vi "Process.vi"(8 "error in":errorcluster, 11 "MAUI":refnum<class "MAUI.lvclass">) -> (0 "error out":errorcluster, 3 "MAUI out":refnum<class "MAUI.lvclass">)   [LabVIEW 2016, in "MAUI.lvclass"]
doc: "---------------------------------------------------------------\nJKI State Machine Objects™\nhttp://jki.net/state-machine-objects/\nCopyright (C) 2005-2015, JKI <info@jki.net>\nALL RIGHTS RESERVEDJKI State Machine Objects (SMO) 1.0.0.5\nJKI - JKI\nCopyright (c) 2016, JKI"
uses:
  MAUI.lvclass
  C:/Program Files (x86)/National Instruments/LabVIEW 2016/vi.lib/JKI/JKI SMO/SMO/SMO.lvclass
  C:/Program Files (x86)/National Instruments/LabVIEW 2016/vi.lib/JKI/JKI SMO/SMO.UI/SMO.UI.lvclass
  <vilib>/JKI/JKI SMO/SMO/Typedefs/Parent Call--Enum.ctl
  MAUI.lvclass/MAUI.ctl
  <vilib>/JKI/JKI SMO/SMO.UI/SMO.UI.lvclass
  <vilib>/JKI/JKI SMO/SMO/SMO.lvclass
panel:
  # "For instructions on how to use the JKI State Machine Objects, examples and video tutorials, visit:\nhttp://jki.net/state-machine-objects/\n\nJKI State Machine Objects™\nhttp://jki.net/state-machine-objects/\nCopyright (C) 2005-2015, JKI <info@jki.net>\nALL RIGHTS RESERVED"
  # "SMO UI Template"
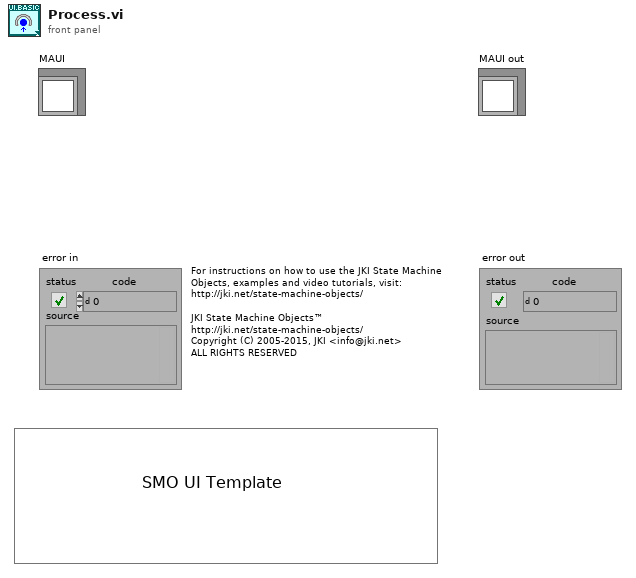
[diagram p1: front panel]
types:
  T1 = typedef "SMO.lvclass/Parent Call--Enum.ctl" = enum16{"Allows parent to run", "Does not request parent to run"}
  T2 = enum32{"invalid app kind", "Development System", "Run Time System", "Student Edition", "Embedded LabVIEW", "Evaluation", "Custom"}
  T3 = enum32{"Invalid", "Standard", "Closed", "Hidden", "Minimized", "Maximized"}
  T4 = typedef "MAUI.lvclass/PrivateEvents--MAUI.Update Left Subpanel.ctl" = i32
  T5 = cluster{"Core":cluster{"Current VI Reference":refnum<vi>, "Close Panel on Exit?":bool, "error":errorcluster}, "Self Reference":refnum<class "MAUI.lvclass">, "Your string data":string}
  T6 = typedef "MAUI.lvclass/PrivateEvents--MAUI.UpdateRightSubpanel.ctl" = i32
  T7 = typedef "MAUI.lvclass/PanelData.ctl" = cluster{"Subpanel":refnum<vi>, "Ring":refnum<vi>, "Active":i32}
  T8 = typedef "MAUI.lvclass/PanelDataNotifier.ctl" = refnum<notifier>
  T9 = cluster{"Subpanel":refnum<vi>, "Ring":refnum<vi>, "Active":i32}
  T10 = cluster{"Current VI Reference":refnum<vi>, "Close Panel on Exit?":bool, "error":errorcluster}
  T11 = typedef "SMO.lvclass/Protected Events.ctl" = cluster{"StopProcesses":refnum<user-event>, "AbortProcesses":refnum<user-event>, "Config Changed":refnum<user-event>, "Dependency":refnum<user-event>}
  T12 = typedef "MAUI.lvclass/PrivateEvents--Cluster.ctl" = cluster{"SetLeftData":refnum<user-event>, "SetRightData":refnum<user-event>, "GetRightData":refnum<user-event>, "GetLeftData":refnum<user-event>, "SetEmbedded":refnum<user-event>, "GetEmbedded":refnum<user-event>, "Update Left Subpanel":refnum<user-event>, "UpdateRightSubpanel":refnum<user-event>}
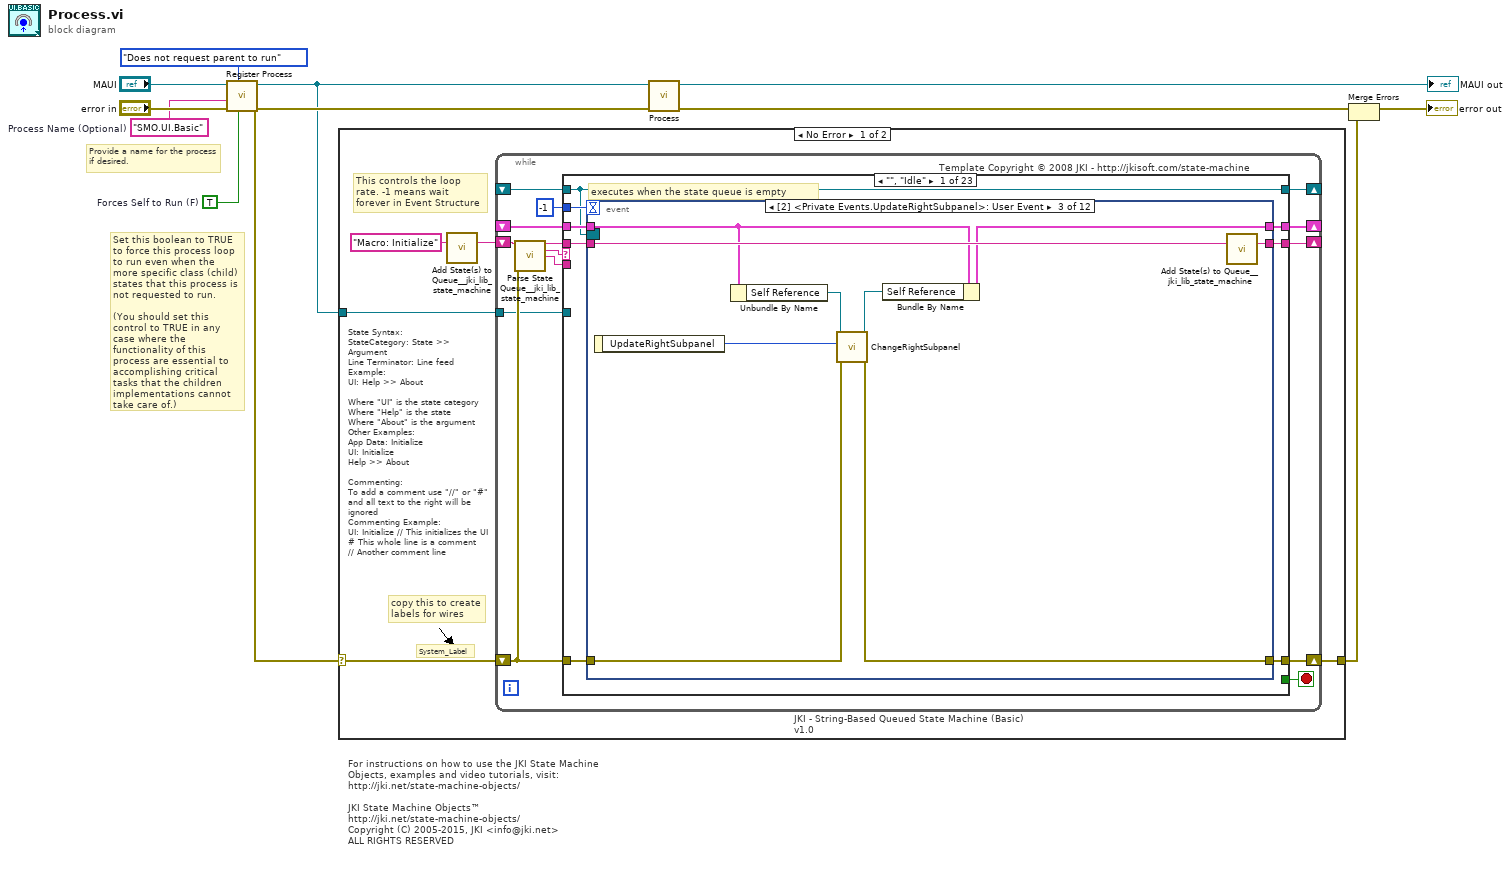
[diagram p0: block diagram]
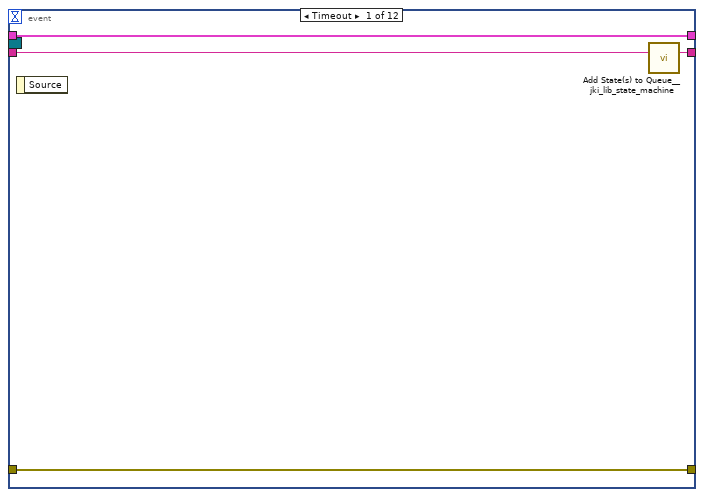
[diagram p2: hidden frame]
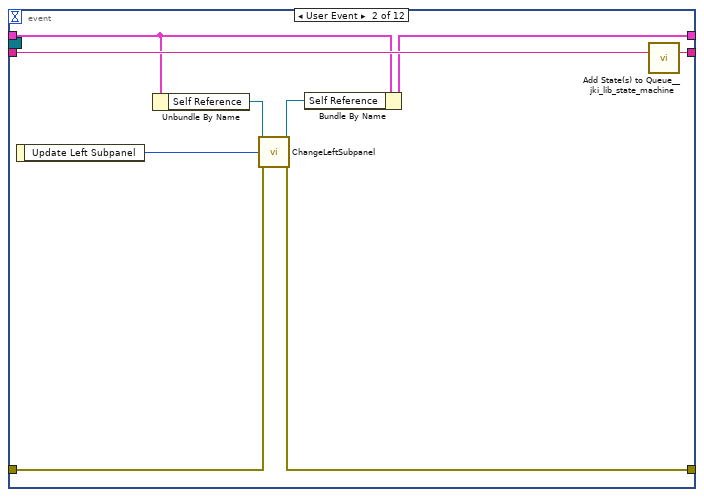
[diagram p3: hidden frame]
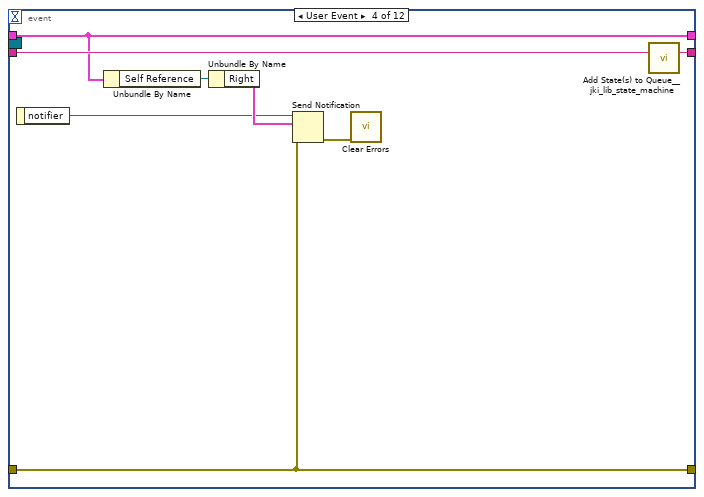
[diagram p4: hidden frame]
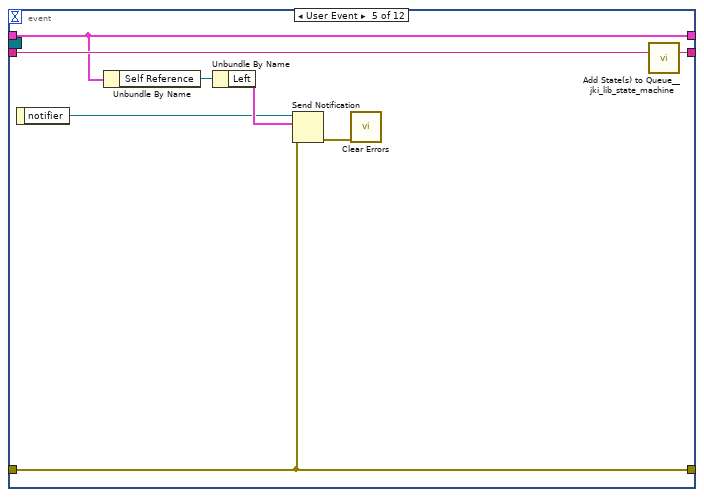
[diagram p5: hidden frame]
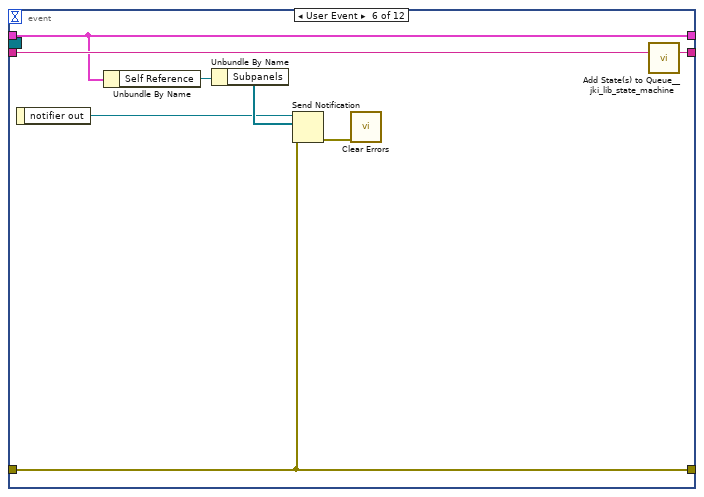
[diagram p6: hidden frame]
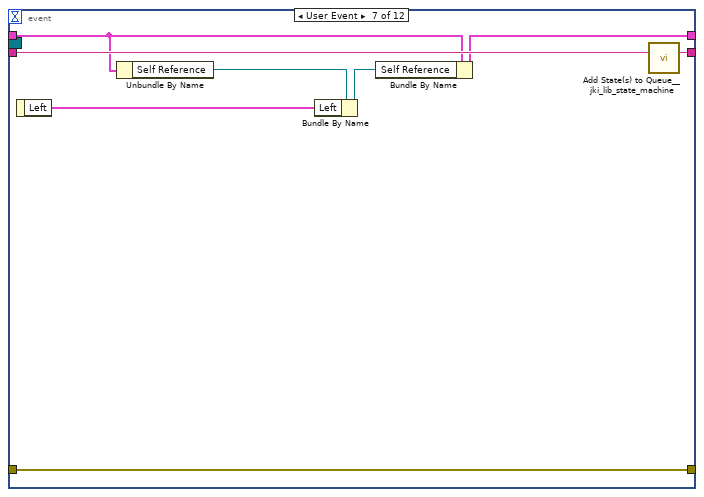
[diagram p7: hidden frame]
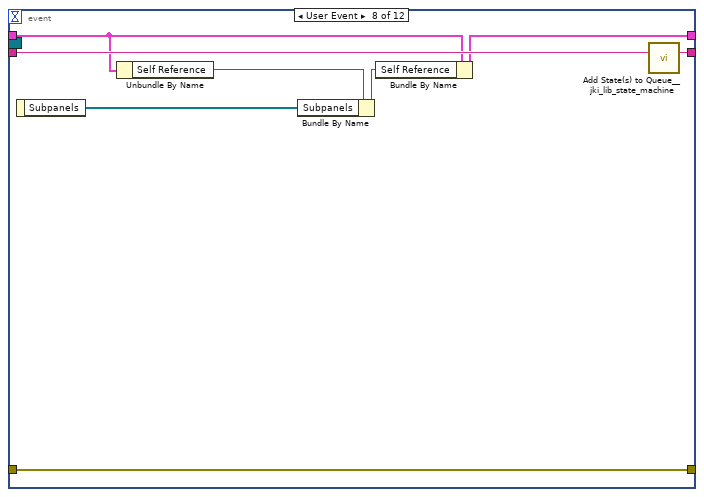
[diagram p8: hidden frame]
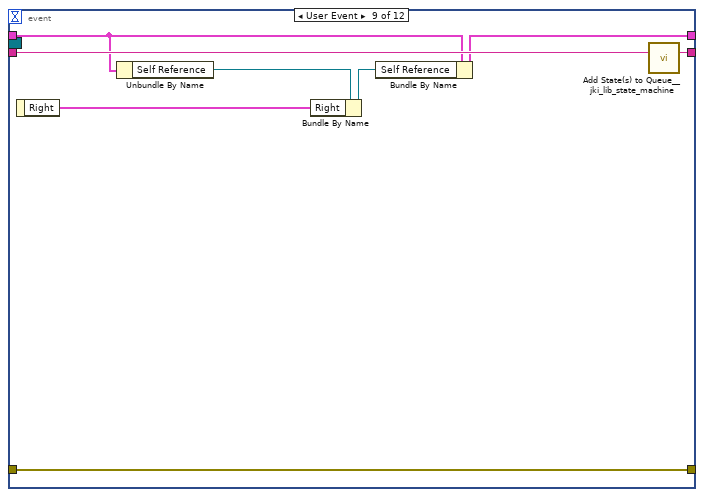
[diagram p9: hidden frame]
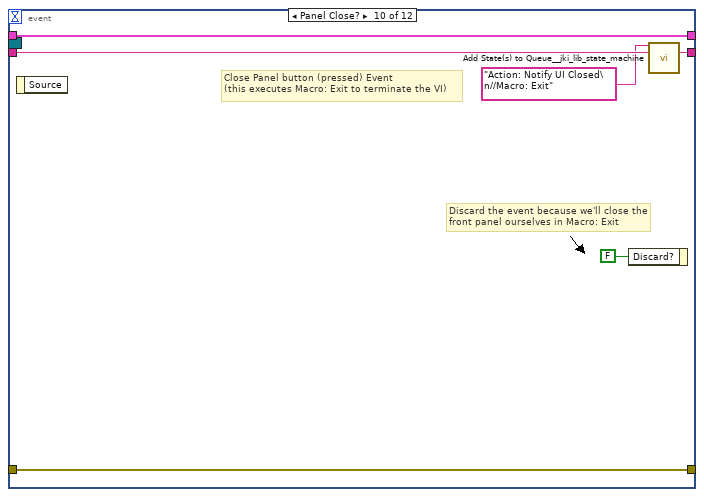
[diagram p10: hidden frame]
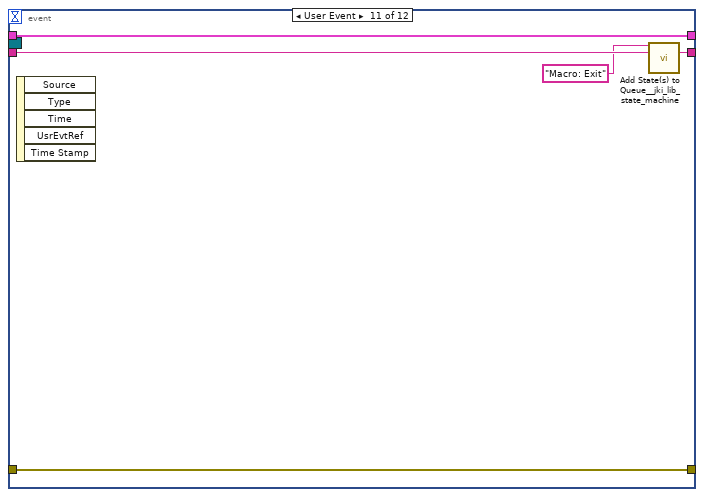
[diagram p11: hidden frame]
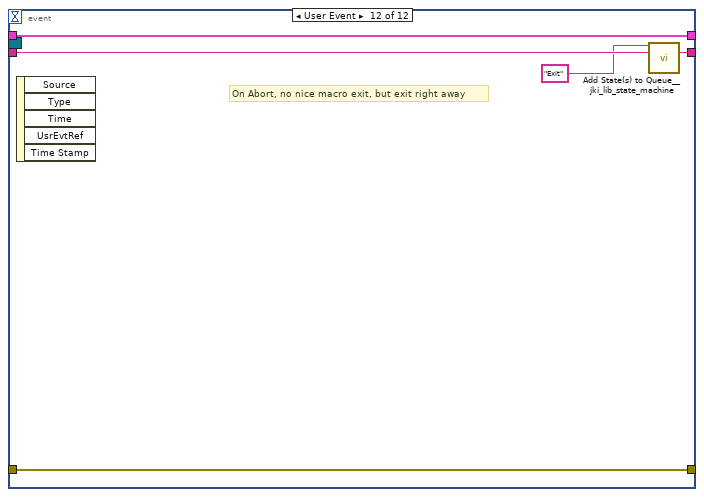
[diagram p12: hidden frame]
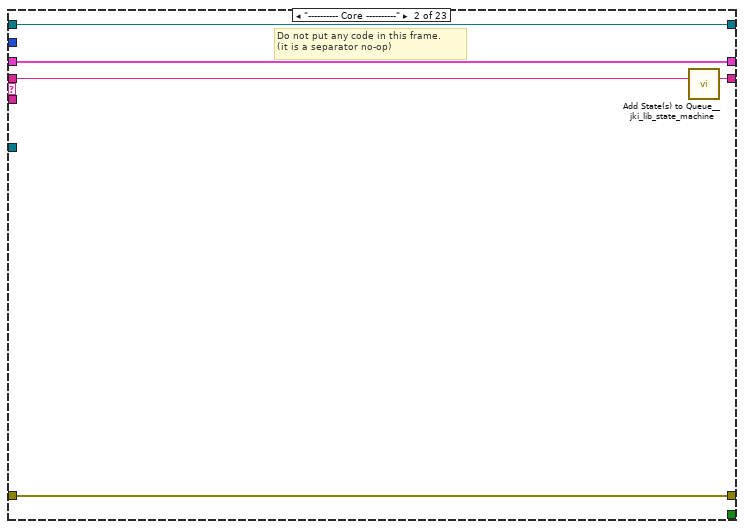
[diagram p13: hidden frame]
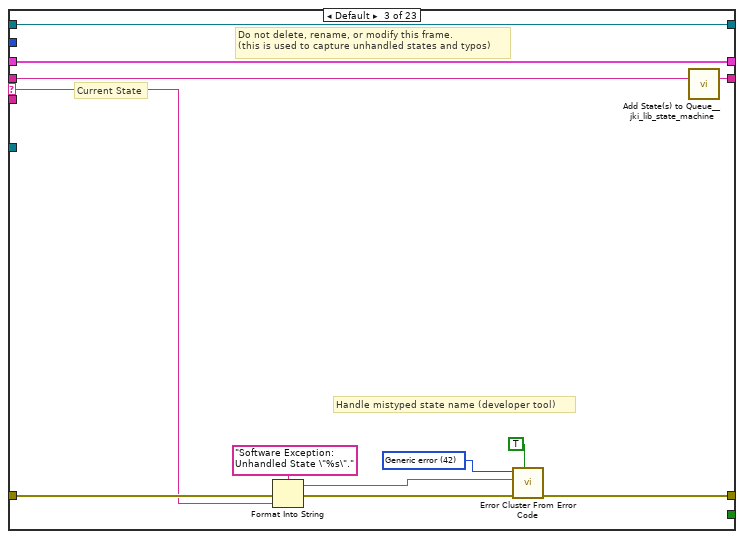
[diagram p14: hidden frame]
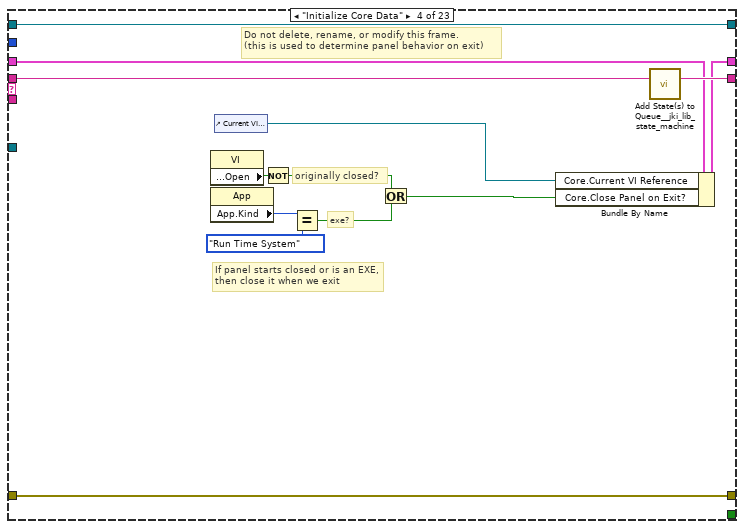
[diagram p15: hidden frame]
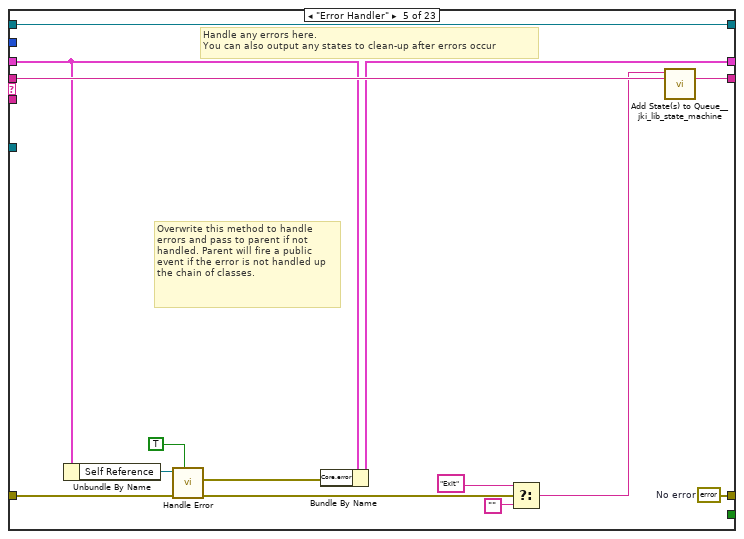
[diagram p16: hidden frame]
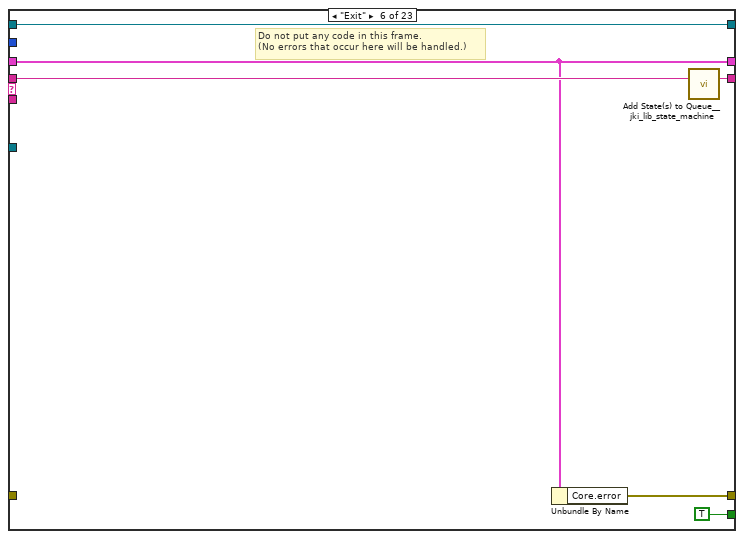
[diagram p17: hidden frame]
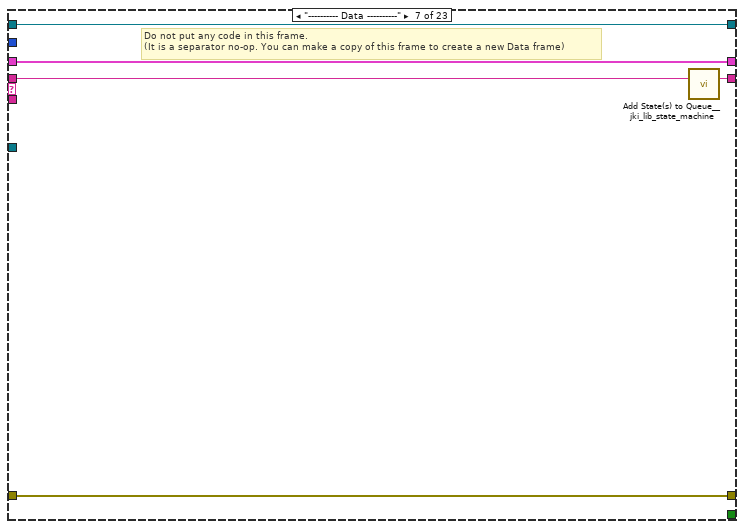
[diagram p18: hidden frame]
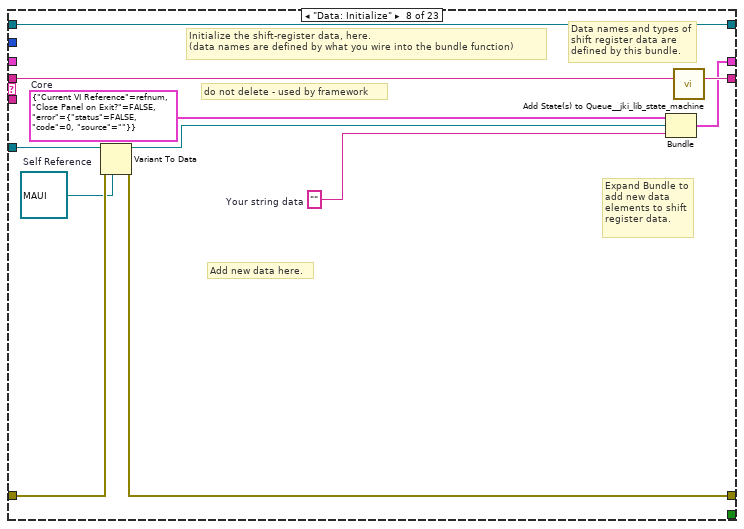
[diagram p19: hidden frame]
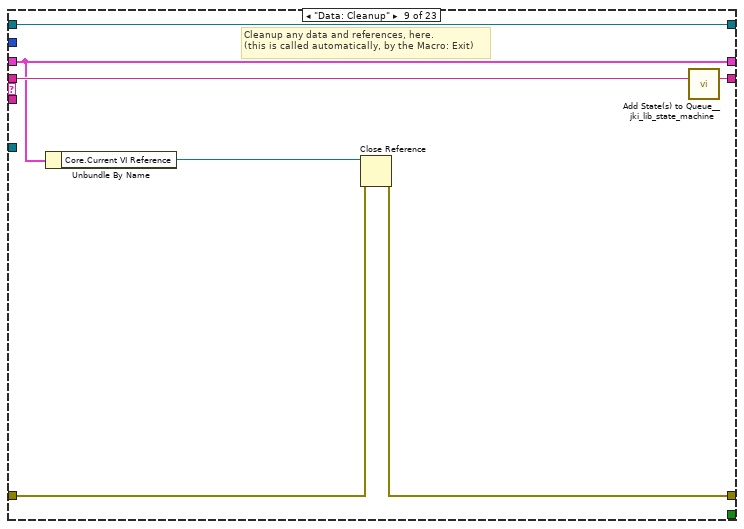
[diagram p20: hidden frame]
diagram:
  w2 = TRUE  # Forces Self to Run (F)
  w1 = "SMO.UI.Basic"  # Process Name (Optional)
  # "Provide a name for the process\nif desired."
  # "Set this boolean to TRUE to force this process loop to run even when the more specific class (child) states that this process is not requested to run.\n\n(You should set this control to TRUE in any case where the functionality of this process are essential to accomplishing critical tasks that the children implementations cannot take care of.)"
  # "For instructions on how to use the JKI State Machine Objects, examples and video tutorials, visit:\nhttp://jki.net/state-machine-objects/\n\nJKI State Machine Objects™\nhttp://jki.net/state-machine-objects/\nCopyright (C) 2005-2015, JKI <info@jki.net>\nALL RIGHTS RESERVED"
  n1 = call <vilib>:"Register Process.vi"("Forces Self to Run (F)"=w2, "Parent Call"=Parent_Call--Enum."Does not request parent to run", "error in (no error)"="error in", "Process Name (optional)"=w1, "SMO"="MAUI") -> ("error out"=w8:errorcluster, "SMO out"=w7:refnum<class "MAUI.lvclass">)  [unwired: 5 in]
  n2 = case shown="No Error" w8 {
    selector: w8 -> [w13 w339]
    tunnel: w7 -> [w14 _]
    tunnel: [w12 w339] -> w4
    frame No Error {
      # "State Syntax:\nStateCategory: State >> Argument\nLine Terminator: Line feed\nExample:\nUI: Help >> About\n\nWhere \"UI\" is the state category\nWhere \"Help\" is the state\nWhere \"About\" is the argument\nOther Examples:\nApp Data: Initialize\nUI: Initialize\nHelp >> About\n\nCommenting:\nTo add a comment use \"//\" or \"#\" and all text to the right will be ignored\nCommenting Example:\nUI: Initialize // This initializes the UI\n# This whole line is a comment\n// Another comment line"
      # "copy this to create labels for wires"
      # "This controls the loop rate. -1 means wait forever in Event Structure"
      # "System_Label"
      n3 = call <vilib>:"Add State(s) to Queue__jki_lib_state_machine.vi"("State(s) in (\"\")"="Macro: Initialize") -> ("States Out"=w16:string)  [unwired: 14 in]
      n4 = while "JKI - String-Based Queued State Machine (Basic) v1.0" {
        shift-right: [w23] -> _
        shift-left: _ -> [w22]
        shift-right: [w26] -> w12
        shift-left: w13 -> [w20]
        shift-right: [w25] -> _
        shift-left: w16 -> [w27]
        tunnel: w14 -> [w19]
        shift-right: [w18] -> _
        shift-left: _ -> [w17]
        stop <- w24 stop-if-true
        # "Template Copyright © 2008 JKI - http://jkisoft.com/state-machine"
        n5 = call <vilib>:"Parse State Queue__jki_lib_state_machine.vi"("State Queue"=w27, "Error In (no error)"=w20) -> ("Remaining States"=w29:string, "Current State"=w30:string, "Arguments"=w28:string)  [unwired: 11 in]
        n6 = case shown="\"\", \"Idle\"" w30 {
          selector: w30 -> [_ _ w131 _ _ _ _ _ _ _ _ _ _ _ _ _ _ _ _ _ _ _ _]
          tunnel: w29 -> [w38 w129 w135 w154 w168 w174 w179 w190 w197 w202 w207 w214 w230 w262 w271 w285 w290 w301 w306 w318 w324 w331 w338]
          tunnel: w28 -> [_ _ _ _ _ _ _ _ _ _ _ w208 w224 _ _ _ _ _ _ _ _ _ _]
          tunnel: w22 -> [w36 w126 w133 w145 w157 w170 w176 _ w192 w199 w205 w212 w226 w259 w267 w276 w287 w298 w303 w316 w322 w327 w334]
          tunnel: [w35 w127 w137 w151 w159 w169 w177 w185 w193 w200 w204 w209 w227 w260 w269 w283 w288 w292 w304 w311 w319 w328 w332] -> w26
          tunnel: w20 -> [w34 w127 w136 w151 w164 _ w177 w186 w194 w200 w204 w210 w228 w260 w269 w283 w288 w293 w304 w313 w320 w328 w333]
          tunnel: [w37 w128 w134 w153 w167 w173 w178 w189 w196 w201 w206 w213 w229 w261 w270 w284 w289 w300 w305 w317 w323 w330 w337] -> w25
          tunnel: [_ _ _ _ _ TRUE _ _ _ _ _ _ _ _ _ _ _ _ _ _ _ _ _] -> w24
          tunnel: [w33 w126 w133 w152 w156 w170 w176 w188 w192 w199 w205 w212 w226 w259 w267 w276 w287 w298 w303 w316 w322 w326 w334] -> w23
          tunnel: -1 ("Timeout") -> [w32 _ _ _ _ _ _ _ _ _ _ _ _ _ _ _ _ _ _ _ _ _ _]
          tunnel: w19 -> [_ _ _ _ _ _ _ w183 _ _ _ _ _ _ _ _ _ _ _ _ _ _ _]
          tunnel: [w31 w125 w130 w142 w166 w171 w175 w181 w191 w198 w203 w211 w223 w258 w268 w277 w286 w299 w302 w315 w321 w329 w336] -> w18
          tunnel: w17 -> [w31 w125 w130 w142 w166 w171 w175 w181 w191 w198 w203 w211 w223 w258 w268 w277 w286 w299 w302 _ w321 w329 w336]
          frame "", "Idle" {
            # "executes when the state queue is empty"
            n7 = event shown="[2] <Private Events.UpdateRightSubpanel>: User Event" {
              selector: w31 -> [_ _ _ _ _ _ _ _ _ _ _ _]
              dyn-events: _ -> [_ _ _ _ _ _ _ _ _ _ _ _]
              timeout: w32 -> [_ _ _ _ _ _ _ _ _ _ _ _]
              tunnel: w38 -> [w42 w51 w60 w68 w76 w84 w92 w100 w108 w114 w119 w124]
              tunnel: [w41 w50 w59 w67 w75 w83 w91 w99 w107 w113 w118 w123] -> w37
              tunnel: w36 -> [w39 w47 w58 w66 w74 w82 w88 w96 w104 w110 w116 w121]
              tunnel: [w40 w43 w52 w62 w70 w78 w90 w98 w106 w109 w117 w122] -> w35
              tunnel: w34 -> [w40 w44 w53 w62 w70 w78 w90 w98 w106 w109 w117 w122]
              tunnel: [w39 w46 w57 w66 w74 w82 w87 w95 w103 w110 w116 w121] -> w33
              event Timeout {
                n8 = event-data() -> ()  [unwired: 1 in, 1 out]
                n9 = call <vilib>:"Add State(s) to Queue__jki_lib_state_machine.vi"("State(s) in (\"\")"=w42) -> ("States Out"=w41:string)  [unwired: 14 in]
              }
              event User Event {
                n10 = event-data() -> ("Update Left Subpanel"=w49:T4)  [unwired: 1 in]
                n11 = Unbundle By Name(w47) -> ("Self Reference"=w48:refnum<class "MAUI.lvclass">)
                n12 = call "ChangeLeftSubpanel.vi"("error in (no error)"=w44, "Left Active"=w49, "MAUI in"=w48) -> ("error out"=w43:errorcluster, "MAUI out"=w45:refnum<class "MAUI.lvclass">)  [unwired: 7 in]
                n13 = Bundle By Name(cluster=w47, "Self Reference"=w45) -> (w46:T5)
                n14 = call <vilib>:"Add State(s) to Queue__jki_lib_state_machine.vi"("State(s) in (\"\")"=w51) -> ("States Out"=w50:string)  [unwired: 14 in]
              }
              event User Event {
                n15 = event-data() -> ("UpdateRightSubpanel"=w54:T6)  [unwired: 1 in]
                n16 = Unbundle By Name(w58) -> ("Self Reference"=w56:refnum<class "MAUI.lvclass">)
                n17 = call "ChangeRightSubpanel.vi"("error in (no error)"=w53, "Left Active"=w54, "MAUI in"=w56) -> ("error out"=w52:errorcluster, "MAUI out"=w55:refnum<class "MAUI.lvclass">)  [unwired: 7 in]
                n18 = Bundle By Name(cluster=w58, "Self Reference"=w55) -> (w57:T5)
                n19 = call <vilib>:"Add State(s) to Queue__jki_lib_state_machine.vi"("State(s) in (\"\")"=w60) -> ("States Out"=w59:string)  [unwired: 14 in]
              }
              event User Event {
                n20 = event-data() -> ("notifier"=w63:refnum<notifier>)  [unwired: 1 in]
                n21 = Unbundle By Name(w66) -> ("Self Reference"=w65:refnum<class "MAUI.lvclass">)
                n22 = Unbundle By Name(w65) -> ("Right"=w64:T7)
                n23 = Send Notification(notification=w64, notifier=w63, error in (no error)=w62) -> (error out=w61:errorcluster)  [unwired: 1 out]
                n24 = call <vilib>:"Clear Errors.vi"("error in (no error)"=w61) -> ()  [unwired: 5 in, 2 out]
                n25 = call <vilib>:"Add State(s) to Queue__jki_lib_state_machine.vi"("State(s) in (\"\")"=w68) -> ("States Out"=w67:string)  [unwired: 14 in]
              }
              event User Event {
                n26 = event-data() -> ("notifier"=w71:T8)  [unwired: 1 in]
                n27 = Unbundle By Name(w74) -> ("Self Reference"=w73:refnum<class "MAUI.lvclass">)
                n28 = Unbundle By Name(w73) -> ("Left"=w72:T7)
                n29 = Send Notification(notification=w72, notifier=w71, error in (no error)=w70) -> (error out=w69:errorcluster)  [unwired: 1 out]
                n30 = call <vilib>:"Clear Errors.vi"("error in (no error)"=w69) -> ()  [unwired: 5 in, 2 out]
                n31 = call <vilib>:"Add State(s) to Queue__jki_lib_state_machine.vi"("State(s) in (\"\")"=w76) -> ("States Out"=w75:string)  [unwired: 14 in]
              }
              event User Event {
                n32 = event-data() -> ("notifier out"=w79:refnum<notifier>)  [unwired: 1 in]
                n33 = Unbundle By Name(w82) -> ("Self Reference"=w81:refnum<class "MAUI.lvclass">)
                n34 = Unbundle By Name(w81) -> ("Subpanels"=w80:refnum<class "EmbeddedSMO.lvclass">[])
                n35 = Send Notification(notification=w80, notifier=w79, error in (no error)=w78) -> (error out=w77:errorcluster)  [unwired: 1 out]
                n36 = call <vilib>:"Clear Errors.vi"("error in (no error)"=w77) -> ()  [unwired: 5 in, 2 out]
                n37 = call <vilib>:"Add State(s) to Queue__jki_lib_state_machine.vi"("State(s) in (\"\")"=w84) -> ("States Out"=w83:string)  [unwired: 14 in]
              }
              event User Event {
                n38 = event-data() -> ("Left"=w85:T9)  [unwired: 1 in]
                n39 = Unbundle By Name(w88) -> ("Self Reference"=w89:refnum<class "MAUI.lvclass">)
                n40 = Bundle By Name(cluster=w89, "Left"=w85) -> (w86:refnum<class "MAUI.lvclass">)
                n41 = Bundle By Name(cluster=w88, "Self Reference"=w86) -> (w87:T5)
                n42 = call <vilib>:"Add State(s) to Queue__jki_lib_state_machine.vi"("State(s) in (\"\")"=w92) -> ("States Out"=w91:string)  [unwired: 14 in]
              }
              event User Event {
                n43 = event-data() -> ("Subpanels"=w93:refnum<class "EmbeddedSMO.lvclass">[])  [unwired: 1 in]
                n44 = Unbundle By Name(w96) -> ("Self Reference"=w97:refnum<class "MAUI.lvclass">)
                n45 = Bundle By Name(cluster=w97, "Subpanels"=w93) -> (w94:refnum<class "MAUI.lvclass">)
                n46 = Bundle By Name(cluster=w96, "Self Reference"=w94) -> (w95:T5)
                n47 = call <vilib>:"Add State(s) to Queue__jki_lib_state_machine.vi"("State(s) in (\"\")"=w100) -> ("States Out"=w99:string)  [unwired: 14 in]
              }
              event User Event {
                n48 = event-data() -> ("Right"=w101:T9)  [unwired: 1 in]
                n49 = Unbundle By Name(w104) -> ("Self Reference"=w105:refnum<class "MAUI.lvclass">)
                n50 = Bundle By Name(cluster=w105, "Right"=w101) -> (w102:refnum<class "MAUI.lvclass">)
                n51 = Bundle By Name(cluster=w104, "Self Reference"=w102) -> (w103:T5)
                n52 = call <vilib>:"Add State(s) to Queue__jki_lib_state_machine.vi"("State(s) in (\"\")"=w108) -> ("States Out"=w107:string)  [unwired: 14 in]
              }
              event Panel Close? {
                # "Discard the event because we'll close the front panel ourselves in Macro: Exit"
                # "Close Panel button (pressed) Event\n(this executes Macro: Exit to terminate the VI)"
                n53 = event-data() -> ()  [unwired: 1 in, 1 out]
                n54 = event-data("Discard?"=FALSE) -> ()  [unwired: 1 in, 1 out]
                n55 = call <vilib>:"Add State(s) to Queue__jki_lib_state_machine.vi"("State(s) in Front (\"\")"="Action: Notify UI Closed\n//Macro: Exit", "State(s) in (\"\")"=w114) -> ("States Out"=w113:string)  [unwired: 13 in]
              }
              event User Event {
                n56 = event-data() -> ()  [unwired: 1 in, 5 out]
                n57 = call <vilib>:"Add State(s) to Queue__jki_lib_state_machine.vi"("State(s) in Front (\"\")"="Macro: Exit", "State(s) in (\"\")"=w119) -> ("States Out"=w118:string)  [unwired: 13 in]
              }
              event User Event {
                # "On Abort, no nice macro exit, but exit right away"
                n58 = event-data() -> ()  [unwired: 1 in, 5 out]
                n59 = call <vilib>:"Add State(s) to Queue__jki_lib_state_machine.vi"("State(s) in Front (\"\")"="Exit", "State(s) in (\"\")"=w124) -> ("States Out"=w123:string)  [unwired: 13 in]
              }
            }
          }
          frame "---------- Core ----------" {
            # "Do not put any code in this frame.\n(it is a separator no-op)"
            n60 = call <vilib>:"Add State(s) to Queue__jki_lib_state_machine.vi"("State(s) in (\"\")"=w129) -> ("States Out"=w128:string)  [unwired: 14 in]
          }
          frame Default {
            w140 = 42 items=["No error", "Argument error", "Memory is full", "Out of zone", "End of file", "File already open", "Generic file I/O error", "File not found", "File permission error", "Disk is full", "Duplicate path", "Too many files open", "System feature not enabled", "Resource file not found", "Cannot add resource", "Resource not found", "Image not found", "Image memory error", "Pen does not exist", "Config type invalid", "Config token not found", "Config parse error", "Config memory error", "Bad external code format", "Bad external code offset", "External code not present", "Null window", "Destroy window error", "Null menu", "Print aborted", "Bad print record", "Print driver error", "Windows error during printing", "Memory error during printing", "Print dialog error", "Generic print error", "Invalid device refnum", "Device not found", "Device parameter error", "Device unit error", "Cannot open device", "Device call aborted", "Generic error", "Cancelled by user", "Object ID too low", "Object ID too high", "Object not in heap", "Unknown heap", "Unknown object (invalid DefProc)", "Unknown object (DefProc not in table)", "Message out of range", "Invalid (null) method", "Unknown message", "Manager call not supported", "Bad address", "Network operation in progress", "Network operation timed out", "Connection is busy", "Network attribute not supported", "Network error", "Address in use", "System out of memory", "Connection aborted", "Connection refused", "Not connected", "Already connected", "Connection closed", "Initialization error (interapplication manager)", "Bad occurrence", "Wait on unbound occurrence handler", "Occurrence queue overflow", "Datalog type conflict", "Unused", "Unrecognized type (interapplication manager)", "Memory corrupt", "Failed to make temporary DLL", "Old CIN version", "Drag socket not found", "Failed to load drop-object", "Failed to register OLE object", "Failed to release OLE object", "Format specifier type mismatch", "Unknown format specifier", "Too few format specifiers", "Too many format specifiers", "Scan failed", "Newer CIN version", "Error converting to variant", "Runtime menu error", "Password tampered", "Variant attribute not found", "Incompatible variant data type", "Event data is not available", "Event Store is not present", "Occurrence is not found", "Event Queue is not created", "Event info is not available", "Refnum passed is NULL", "Error retrieving Class GUID", "Error retrieving CoClass GUID", "Error retrieving TypeLib GUID.", "Bad built application magic bytes.", "Specific driver is different from the specific driver associated with the Logical Name.", "There is no session opened to the class driver.", "Max Error", "MAX - Error with config objects", "MAX - Error loading configuration", "MAX - Group not supported"]
            # "Current State"
            # "Do not delete, rename, or modify this frame.\n(this is used to capture unhandled states and typos)"
            # "Handle mistyped state name (developer tool)"
            n61 = Format Into String(format string="Software Exception: Unhandled State \"%s\"." ("message"), error in=w136, w131) -> (resulting string=w139:string, error out=w138:errorcluster)  [unwired: 1 in]
            n62 = call <vilib>:"Error Cluster From Error Code.vi"("show call chain? (False)"=TRUE, "error in (no error)"=w138, "error message (\"\")"=w139, "error code (0)"=w140) -> ("error out"=w137:errorcluster)  [unwired: 5 in]
            n63 = call <vilib>:"Add State(s) to Queue__jki_lib_state_machine.vi"("State(s) in (\"\")"=w135) -> ("States Out"=w134:string)  [unwired: 14 in]
          }
          frame "Initialize Core Data" {
            # "Do not delete, rename, or modify this frame.\n(this is used to determine panel behavior on exit)"
            # "originally closed?"
            # "exe?"
            # "If panel starts closed or is an EXE, then close it when we exit"
            n64 = property class="VI"() -> ("Front Panel.Open"=w150:bool)  [unwired: 2 in, 2 out]
            n65 = property class="App"() -> ("App.Kind"=w149:T2)  [unwired: 2 in, 2 out]
            n66 = control-ref of="Current VI Reference"() -> (w143:refnum<vi>)
            n67 = Not(x=w150) -> (.not. x?=w147:bool)
            n68 = Equal?(x=w149, y=T2."Run Time System" ("Application:Kind")) -> (x = y?=w146:bool)
            n69 = Or(x=w147, y=w146) -> (x .or. y?=w144:bool)
            n70 = Bundle By Name(cluster=w145, "Core.Current VI Reference"=w143, "Core.Close Panel on Exit?"=w144) -> (w152:T5)
            n71 = call <vilib>:"Add State(s) to Queue__jki_lib_state_machine.vi"("State(s) in (\"\")"=w154) -> ("States Out"=w153:string)  [unwired: 14 in]
          }
          frame "Error Handler" {
            w159 = errorcluster {"status"=FALSE, "code"=0, "source"=""}  # No error
            # "Overwrite this method to handle errors and pass to parent if not handled. Parent will fire a public event if the error is not handled up the chain of classes."
            # "Handle any errors here.\nYou can also output any states to clean-up after errors occur"
            n72 = Unbundle By Name(w157) -> ("Self Reference"=w165:refnum<class "MAUI.lvclass">)
            n73 = call-dynamic "Handle Error.vi"("Stop on Unhandled Error (T)"=TRUE, "error in"=w164, "SMO"=w165) -> ("handling error"=w160:errorcluster, "Unhandled error"=w158:errorcluster)  [unwired: 6 in, 1 out]
            n74 = Bundle By Name(cluster=w157, "Core.error"=w158) -> (w156:T5)
            n75 = Select(t="Exit", s=w160, f="") -> (s? t:f=w161:string)
            n76 = call <vilib>:"Add State(s) to Queue__jki_lib_state_machine.vi"("State(s) in Front (\"\")"=w161, "State(s) in (\"\")"=w168) -> ("States Out"=w167:string)  [unwired: 13 in]
          }
          frame "Exit" {
            # "Do not put any code in this frame.\n(No errors that occur here will be handled.)"
            n77 = Unbundle By Name(w170) -> ("Core.error"=w169:errorcluster)
            n78 = call <vilib>:"Add State(s) to Queue__jki_lib_state_machine.vi"("State(s) in (\"\")"=w174) -> ("States Out"=w173:string)  [unwired: 14 in]
          }
          frame "---------- Data ----------" {
            # "Do not put any code in this frame.\n(It is a separator no-op. You can make a copy of this frame to create a new Data frame)"
            n79 = call <vilib>:"Add State(s) to Queue__jki_lib_state_machine.vi"("State(s) in (\"\")"=w179) -> ("States Out"=w178:string)  [unwired: 14 in]
          }
          frame "Data: Initialize" {
            w180 = T10 {"Current VI Reference"=refnum, "Close Panel on Exit?"=FALSE, "error"={"status"=FALSE, "code"=0, "source"=""}}  # Core
            w184 = refnum<class "MAUI.lvclass"> refnum  # Self Reference
            w187 = ""  # Your string data
            # "do not delete - used by framework"
            # "Expand Bundle to add new data elements to shift register data."
            # "Add new data here."
            # "Data names and types of shift register data are defined by this bundle."
            # "Initialize the shift-register data, here.\n(data names are defined by what you wire into the bundle function)"
            n80 = Variant To Data(error in=w186, type=w184, Variant=w183) -> (data=w182:refnum<class "MAUI.lvclass">, error out=w185:errorcluster)
            n81 = Bundle("Core"=w180, "Self Reference"=w182, "Your string data"=w187) -> (w188:T5)  [unwired: 1 in]
            n82 = call <vilib>:"Add State(s) to Queue__jki_lib_state_machine.vi"("State(s) in (\"\")"=w190) -> ("States Out"=w189:string)  [unwired: 14 in]
          }
          frame "Data: Cleanup" {
            # "Cleanup any data and references, here.\n(this is called automatically, by the Macro: Exit)"
            n83 = Unbundle By Name(w192) -> ("Core.Current VI Reference"=w195:refnum<vi>)
            n84 = Close Reference(reference=w195, error in (no error)=w194) -> (error out=w193:errorcluster)
            n85 = call <vilib>:"Add State(s) to Queue__jki_lib_state_machine.vi"("State(s) in (\"\")"=w197) -> ("States Out"=w196:string)  [unwired: 14 in]
          }
          frame "---------- UI ----------" {
            # "Do not put any code in this frame.\n(It is a separator no-op. You can make a copy of this frame to create a new UI frame)"
            n86 = call <vilib>:"Add State(s) to Queue__jki_lib_state_machine.vi"("State(s) in (\"\")"=w202) -> ("States Out"=w201:string)  [unwired: 14 in]
          }
          frame "UI: Initialize" {
            # "Initialize the User Interface, here.\n(this is called automatically, by the Macro: Init)"
            n87 = call <vilib>:"Add State(s) to Queue__jki_lib_state_machine.vi"("State(s) in (\"\")"=w207) -> ("States Out"=w206:string)  [unwired: 14 in]
          }
          frame "UI: Cursor Set" {
            # "Argument"
            # "Initialize the User Interface, here.\n(this is called automatically, by the Macro: Init)"
            n88 = disable-structure shown="Default" {
              disable-tunnel: w210 -> [w215 w218]
              disable-tunnel: [w215 w217] -> w209
              disable-tunnel: w208 -> [_ w216]
              frame condition #0 {
              }
              frame condition #1 (active) {
                n89 = case shown="\"Idle\", Default" w216 {
                  tunnel: w218 -> [w220 w222]
                  tunnel: [w219 w221] -> w217
                  frame "Idle", Default {
                    n90 = call <vilib>:"Unset Busy.vi"("error in (no error)"=w220) -> ("error out"=w219:errorcluster)  [unwired: 10 in]
                  }
                  frame "Busy" {
                    n91 = call <vilib>:"Set Busy.vi"("error in (no error)"=w222) -> ("error out"=w221:errorcluster)  [unwired: 9 in, 1 out]
                  }
                }
              }
            }
            n92 = call <vilib>:"Add State(s) to Queue__jki_lib_state_machine.vi"("State(s) in (\"\")"=w214) -> ("States Out"=w213:string)  [unwired: 14 in]
          }
          frame "UI: Front Panel State" {
            # "Argument"
            # "Set Front Panel Open or Closed\n(Usage: \"UI: Front Panel State >> Open|Close\")"
            n93 = Unbundle By Name(w226) -> ("Core.Current VI Reference"=w225:refnum<vi>)
            n94 = disable-structure shown="Default" {
              disable-tunnel: w228 -> [w234 w257]
              disable-tunnel: [w233 w257] -> w227
              disable-tunnel: w225 -> [w232 _]
              disable-tunnel: w224 -> [w231 _]
              frame condition #0 (active) {
                n95 = case shown="\"Close\"" w231 {
                  tunnel: w234 -> [w238 w251]
                  tunnel: [w240 w252] -> w233
                  tunnel: w232 -> [w239 w249]
                  frame "Open", Default {
                    n96 = property class="VI"(reference=w239, error in=w238) -> (reference out=w236:refnum<vi>, error out=w237:errorcluster, "FP.State"=w235:T3)
                    n97 = case shown="\"Closed\"" w235 {
                      tunnel: [w243 w246] -> w240
                      tunnel: w237 -> [w242 w246]
                      tunnel: w236 -> [w241 _]
                      frame "Closed" {
                        n98 = invoke class="VI" method="FP.Open"(reference=w241, error in=w242, "Activate"=TRUE, "State"=T3."Standard") -> (error out=w243:errorcluster)  [unwired: 1 in, 4 out]
                      }
                      frame Default {
                      }
                    }
                  }
                  frame "Close" {
                    n99 = property class="VI"(reference=w249, error in=w251) -> (reference out=w248:refnum<vi>, error out=w250:errorcluster, "FP.State"=w247:T3)
                    n100 = case shown="Default" w247 {
                      tunnel: [w253 w256] -> w252
                      tunnel: w250 -> [w253 w255]
                      tunnel: w248 -> [_ w254]
                      frame "Invalid", "Closed" {
                      }
                      frame Default {
                        n101 = invoke class="VI" method="FP.Close"(reference=w254, error in=w255) -> (error out=w256:errorcluster)  [unwired: 1 in, 2 out]
                      }
                    }
                  }
                }
              }
              frame condition #1 {
              }
            }
            n102 = call <vilib>:"Add State(s) to Queue__jki_lib_state_machine.vi"("State(s) in (\"\")"=w230) -> ("States Out"=w229:string)  [unwired: 14 in]
          }
          frame "---------- Macro ----------" {
            # "Do not put any code in this frame.\n(It is a separator no-op. You can make a copy of this frame to create a new Macro frame)"
            n103 = call <vilib>:"Add State(s) to Queue__jki_lib_state_machine.vi"("State(s) in (\"\")"=w262) -> ("States Out"=w261:string)  [unwired: 14 in]
          }
          frame "Macro: Initialize" {
            w265 = "UI: Initialize\n//UI: Front Panel State >> Open"  # UI: Initialize //UI: Front Panel State >> Open
            # "Initialization Macro\n(This is called once, when the VI starts)"
            n104 = call <vilib>:"Add State(s) to Queue__jki_lib_state_machine.vi"("State(s) in Front (\"\")"="Data: Initialize\nInitialize Core Data\nEvents: Register", "State(s) in (\"\")"="Process: Sync", "State(s) at Back (\"\")"=w265) -> ("States Out"=w264:string)  [unwired: 12 in]
            n105 = call <vilib>:"Add State(s) to Queue__jki_lib_state_machine.vi"("State(s) in Front (\"\")"=w264, "State(s) in (\"\")"=w271) -> ("States Out"=w270:string)  [unwired: 13 in]
          }
          frame "Macro: Exit" {
            # "Exit Macro\n(This is called once, when the VI exits)"
            n106 = Unbundle By Name(w276) -> ("Core.Close Panel on Exit?"=w282:bool)
            n107 = Select(t="//UI: Front Panel State >> Close", s=w282, f="") -> (s? t:f=w279:string)
            n108 = call <vilib>:"Add State(s) to Queue__jki_lib_state_machine.vi"("State(s) in Front (\"\")"="Data: Cleanup\nEvents: Unregister", "State(s) in (\"\")"="Process: Sync", "State(s) at Back (\"\")"="Exit") -> ("States Out"=w273:string)  [unwired: 12 in]
            n109 = call <vilib>:"Add State(s) to Queue__jki_lib_state_machine.vi"("State(s) in (\"\")"=w279, "State(s) at Back (\"\")"=w273) -> ("States Out"=w278:string)  [unwired: 13 in]
            n110 = call <vilib>:"Add State(s) to Queue__jki_lib_state_machine.vi"("State(s) in Front (\"\")"=w278, "State(s) in (\"\")"=w285) -> ("States Out"=w284:string)  [unwired: 13 in]
          }
          frame "---------- Process ----------" {
            # "Template Separator\n(You can make a copy of, or modify, this frame)"
            n111 = call <vilib>:"Add State(s) to Queue__jki_lib_state_machine.vi"("State(s) in (\"\")"=w290) -> ("States Out"=w289:string)  [unwired: 14 in]
          }
          frame "Process: Sync" {
            n112 = Unbundle By Name(w298) -> ("Self Reference"=w294:refnum<class "MAUI.lvclass">)
            n113 = call <vilib>:"WaitOnProcessSync.vi"("error in (no error)"=w293, "SMO"=w294) -> ("error out"=w292:errorcluster, "Don't run?"=w297:bool)  [unwired: 7 in, 1 out]
            n114 = Select(t="Data: Cleanup\nEvents: Unregister\nExit", s=w297, f="") -> (s? t:f=w291:string)
            n115 = call <vilib>:"Add State(s) to Queue__jki_lib_state_machine.vi"("State(s) in Front (\"\")"=w291, "State(s) in (\"\")"=w301) -> ("States Out"=w300:string)  [unwired: 13 in]
          }
          frame "---------- Events ----------" {
            # "Template Separator\n(You can make a copy of, or modify, this frame)"
            n116 = call <vilib>:"Add State(s) to Queue__jki_lib_state_machine.vi"("State(s) in (\"\")"=w306) -> ("States Out"=w305:string)  [unwired: 14 in]
          }
          frame "Events: Register" {
            # "Expand to add\nmore events"
            # "Base Class Protected Events"
            n117 = Unbundle By Name(w316) -> ("Self Reference"=w309:refnum<class "MAUI.lvclass">)
            n118 = call <vilib>:"GetProtectedEvents.vi"("SMO"=w309) -> ("error out"=w310:errorcluster, "SMO Protected Events"=w314:T11)  [unwired: 8 in, 1 out]
            n119 = call "MAUI.GetPrivateEvents.vi"("MAUI"=w309) -> ("error out"=w307:errorcluster, "Private Events"=w308:T12)  [unwired: 8 in, 1 out]
            n120 = register-events(w314, w308) -> (reference out=w315:refnum<event-registration>, error out=w312:errorcluster)  [unwired: 2 in]
            n121 = Merge Errors(w313, w312, w310, w307) -> (w311:errorcluster)
            n122 = call <vilib>:"Add State(s) to Queue__jki_lib_state_machine.vi"("State(s) in (\"\")"=w318) -> ("States Out"=w317:string)  [unwired: 14 in]
          }
          frame "Events: Unregister" {
            n123 = Unregister For Events(event registration refnum=w321, error in=w320) -> (error out=w319:errorcluster)
            n124 = call <vilib>:"Add State(s) to Queue__jki_lib_state_machine.vi"("State(s) in (\"\")"=w324) -> ("States Out"=w323:string)  [unwired: 14 in]
          }
          frame "---------- Action ----------" {
            n125 = Unbundle By Name(w327) -> ("Self Reference"=w325:refnum<class "MAUI.lvclass">)
            n126 = Bundle By Name(cluster=w327, "Self Reference"=w325) -> (w326:T5)
            n127 = call <vilib>:"Add State(s) to Queue__jki_lib_state_machine.vi"("State(s) in (\"\")"=w331) -> ("States Out"=w330:string)  [unwired: 14 in]
          }
          frame "Action: Notify UI Closed" {
            # "Notify that the UI has been closed"
            n128 = Unbundle By Name(w334) -> ("Self Reference"=w335:refnum<class "MAUI.lvclass">)
            n129 = call <vilib>:"Hide.vi"("error in (no error)"=w333, "SMO.UI"=w335) -> ("error out"=w332:errorcluster)  [unwired: 8 in, 1 out]
            n130 = call <vilib>:"Add State(s) to Queue__jki_lib_state_machine.vi"("State(s) in (\"\")"=w338) -> ("States Out"=w337:string)  [unwired: 14 in]
          }
        }
      }
    }
    frame Error {
    }
  }
  n131 = call-parent "Process.vi"("error in (no error)"=w8, "SMO.UI"=w7) -> ("error out"=w5:errorcluster, "SMO.UI out"=→"MAUI out":refnum<class "MAUI.lvclass">)  [unwired: 8 in]
  n132 = Merge Errors(w5, w4) -> (→"error out":errorcluster)
